vi "Write Data.vi"(8 "Error In":errorcluster, 10 "Data":u8[](array[numeric]), 11 "LINX Resource":T1) -> (0 "Error Out":errorcluster, 3 "LINX Resource":T1)   [LabVIEW 2013, in "LVH-LINX.lvlib" / "SSD1306.lvlib"]
doc: "Write display data to the SSD1306's graphic memory."
uses:
  SSD1306.lvlib
  Private/Type Defs/LINX Ref.ctl
  Private/Type Defs/Platform.ctl
  Private/Type Defs/Interface.ctl
  Private/Device/Type Defs/LINX Device Config.ctl
  Private/Device/Type Defs/TCP Config.ctl
  Private/Type Defs/Device Family.ctl
  Private/Device/Type Defs/Channels.ctl
  Private/SSD1306 FGV State.ctl
  Peripherals/Digital/Digital Write 1 Chan.vi
  LVH-LINX.lvlib
  Private/Device/Device.lvlib
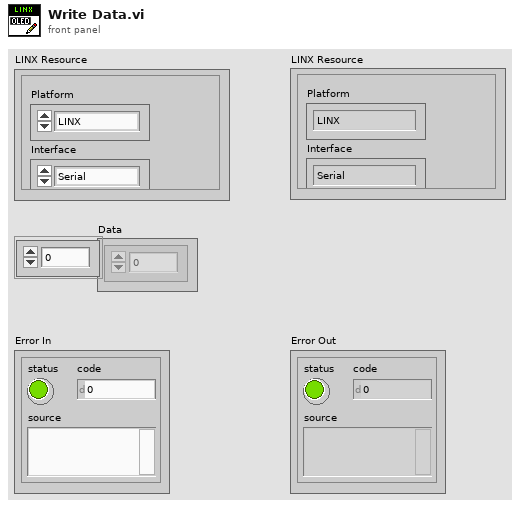
[diagram p1: front panel]
types:
  T1 = typedef "LVH-LINX.lvlib/LINX Ref.ctl" = cluster{"Platform":T2, "Interface":T3, "LINX Device Config":T4}
  T2 = typedef "LVH-LINX.lvlib/Platform.ctl" = enum16{"LINX", "myRIO"}
  T3 = typedef "LVH-LINX.lvlib/Interface.ctl" = enum16{"Serial", "TCP"}
  T4 = typedef "LVH-LINX.lvlib/Device.lvlib/LINX Device Config.ctl" = cluster{"Interface":T3, "COM Port":refnum<visa-resource-name>, "TCP Configuration":T5, "Device Family":T6, "Device ID":u8, "Device Name":string, "TCP Ref":refnum<k5>, "Channels":T7}
  T5 = typedef "LVH-LINX.lvlib/Device.lvlib/TCP Config.ctl" = cluster{"IP Address":string, "Port":u16}
  T6 = typedef "LVH-LINX.lvlib/Device Family.ctl" = enum8{"National Instruments", "Digilent", "Arduino"}
  T7 = typedef "LVH-LINX.lvlib/Channels.ctl" = cluster{"DI Channels":u8[], "DO Channels":u8[], "AI":u8[], "AO":u8[], "PWM":u8[], "QE":u8[], "UART":u8[], "I2C 2":u8[], "SPI":u8[], "CAN":u8[], "AI Ref (V)":dbl, "AO Resolution (Bits)":u8, "AO Ref (V)":dbl}
  T8 = typedef "LVH-LINX.lvlib/SSD1306.lvlib/SSD1306 FGV State.ctl" = enum16{"Init", "Set", "Get"}
  T9 = typedef "LVH-LINX.lvlib/SSD1306.lvlib/SSD1306 Config.ctl" = cluster{"SPI Channel (0)":u8, "VDD Channel":u8, "VBAT Channel":u8, "RESET Channel":u8, "DC Channel":u8, "SPI CS (3)":u8}
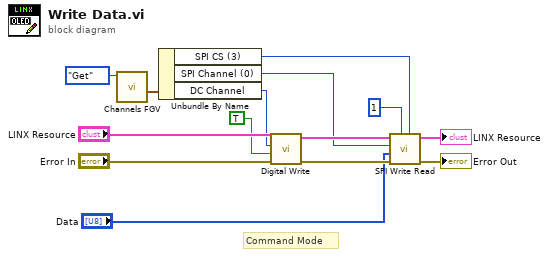
[diagram p0: block diagram]
diagram:
  # "Command Mode"
  n1 = call "Channels FGV.vi"("SSD1306 FGV State"=SSD1306_FGV_State."Get") -> ("SSD1306 Channels"=w11:T9)  [unwired: 10 in]
  n2 = Unbundle By Name(w11) -> ("SPI CS (3)"=w1:u8, "SPI Channel (0)"=w6:u8, "DC Channel"=w10:u8)
  n3 = call-poly "Digital Write.vi"("Error In"="Error In", "Output Value"=TRUE, "DO Channel"=w10, "LINX Resource"="LINX Resource") -> ("Error Out"=w7:errorcluster, "LINX Resource"=w8:T1)  [unwired: 6 in]
  n4 = call "SPI Write Read.vi"("CS Pin (10)"=w1, "SPI Frame Size"=u8 1, "Error In"=w7, "Data"="Data", "SPI Channel (0)"=w6, "LINX Resource"=w8) -> ("Error Out"=→"Error Out":errorcluster, "LINX Resource"=→"LINX Resource":T1)  [unwired: 3 in, 1 out]
